vi "ConditionData_ArrayofLabelsStrings.vi"(8 "error in (no error)":errorcluster, 11 "Condition Data":variant[](array[variant])=[variant(i32 122), variant(i32[] [12, 23])]) -> (0 "error out":errorcluster, 2 "Value":string[](array[string]), 3 "Label":string[](array[string]))   [LabVIEW 2014, in "TableLogger_SQLite_Actor.lvlib" / "TableLogger_SQLite_Actor.lvclass"]
uses:
  TableLogger_SQLite_Actor.lvclass
  TableLogger_Actor/TableLogger_Actor/TableLogger_Actor.lvclass
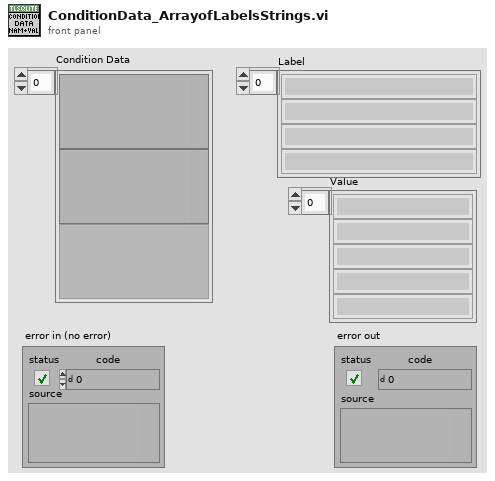
[diagram p1: front panel]
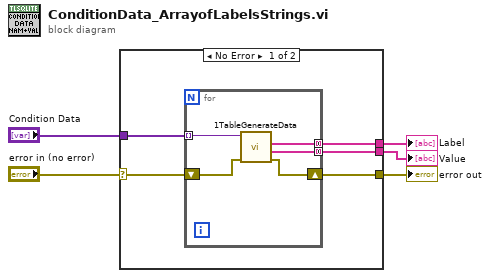
[diagram p0: block diagram]
diagram:
  n1 = case shown="No Error" "error in (no error)" {
    selector: "error in (no error)" -> [w6 w16]
    tunnel: [w10 _] -> w5
    tunnel: [w9 _] -> w4
    tunnel: [w8 w16] -> w3
    tunnel: "Condition Data" -> [w7 _]
    frame No Error {
      n2 = for {
        tunnel: w7 -> [w15] mode=indexing
        tunnel: [w14] -> w10 mode=concatenating
        tunnel: [w13] -> w9 mode=concatenating
        shift-right: [w11] -> w8
        shift-left: w6 -> [w12]
        n3 = call "1TableGenerateData.vi"("error in (no error)"=w12, "Cluster Variant"=w15) -> ("error out"=w11:errorcluster, "Data"=w13:string[], "Headers"=w14:string[])  [unwired: 5 in, 2 out]
      }
    }
    frame Error {
    }
  }
  "Value" <- w4
  "Label" <- w5
  "error out" <- w3
